vi "GenerateAndWriteSignal.vi"() -> ()   [LabVIEW 2025]
uses:
  wfm-type.ctl
panel:
  out "error out":errorcluster
  out "file path out":path
  in  "stop":bool
  in  "wfm type":T1
  in  "frequency":dbl=1e-06 min=1e-06
  in  "amplitude":dbl
  in  "noise RMS":dbl=1.0 format="%.2p"
  in  "#s":dbl=1.0 min=1.0
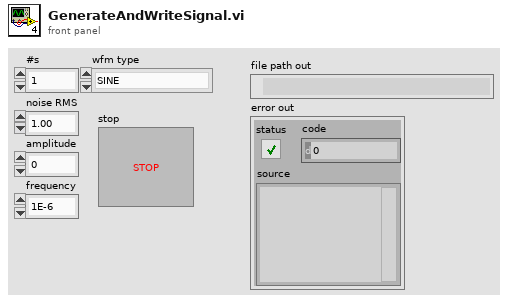
[diagram p1: front panel]
types:
  T1 = typedef "wfm-type.ctl" = enum16{"SINE", "SQUARE", "TRIANGLE", "SAWTOOTH"}
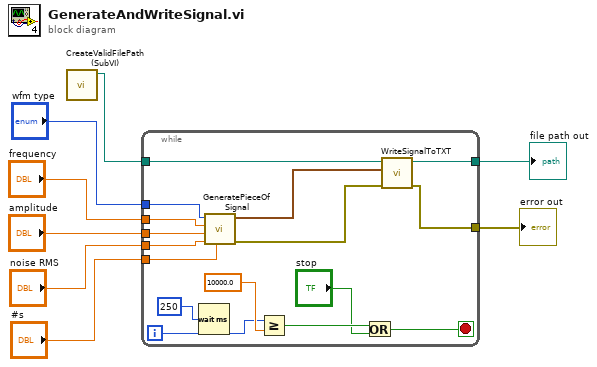
[diagram p0: block diagram]
diagram:
  n1 = call "CreateValidFilePath (SubVI).vi"() -> ("path"=w3:path)  [unwired: 11 in]
  n2 = while {
    tunnel: "#s" -> [w24]
    tunnel: "noise RMS" -> [w23]
    tunnel: "amplitude" -> [w22]
    tunnel: "frequency" -> [w21]
    tunnel: "wfm type" -> [w20]
    tunnel: w3 -> [w16]
    tunnel: [w15] -> w2
    tunnel: [w9] -> w1
    i -> [w13]
    stop <- w10 stop-if-true
    n3 = Wait (ms)(milliseconds to wait=u32 250) -> ()  [unwired: 1 out]
    n4 = call "GeneratePieceOfSignal.vi"("#s"=w24, "noise RMS"=w23, "amplitude"=w22, "frequency"=w21, "wfm type"=w20) -> ("error out"=w17:errorcluster, "wfm out"=w18:waveform(dbl))  [unwired: 5 in]
    n5 = Greater Or Equal?(x=w13, y=10000.0) -> (x >= y?=w12:bool)
    n6 = Or(x=w12, y="stop") -> (x .or. y?=w10:bool)
    n7 = call "WriteSignalToTXT.vi"("error in"=w17, "signal in"=w18, "file path in"=w16) -> ("error out"=w9:errorcluster, "file path out"=w15:path)  [unwired: 7 in]
  }
  "file path out" <- w2
  "error out" <- w1
